vi "LogToFile.vi"(0 "EventData in":T1, 11 "Error In":errorcluster) -> (4 "EventData out":T1, 15 "Error Out":errorcluster)   [LabVIEW 2021, in "Event Logger.lvlib"]
uses:
  Event Logger.lvlib
  TypeDef/EventDataCluster.ctl
  TypeDef/EventValues.ctl
  Migrator/Migrator Reusables/Migrator Reusables.lvlib
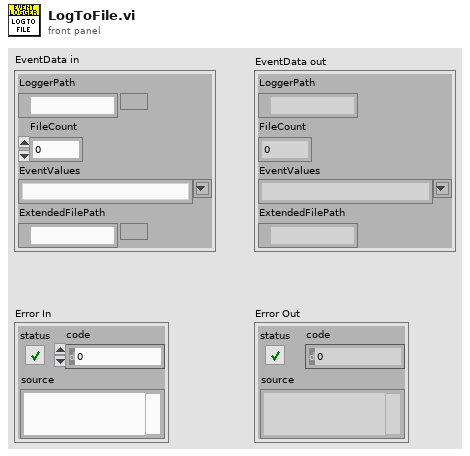
[diagram p1: front panel]
types:
  T1 = typedef "Event Logger.lvlib/EventDataCluster.ctl" = cluster{"LoggerPath":path, "FileCount":i32, "EventValues":T2, "ExtendedFilePath":path}
  T2 = typedef "Event Logger.lvlib/EventValues.ctl" = string
  T3 = typedef "Migrator Reusables.lvlib/ErrorInformation.ctl" = cluster{"Subroutine":string, "ErrorData":errorcluster}
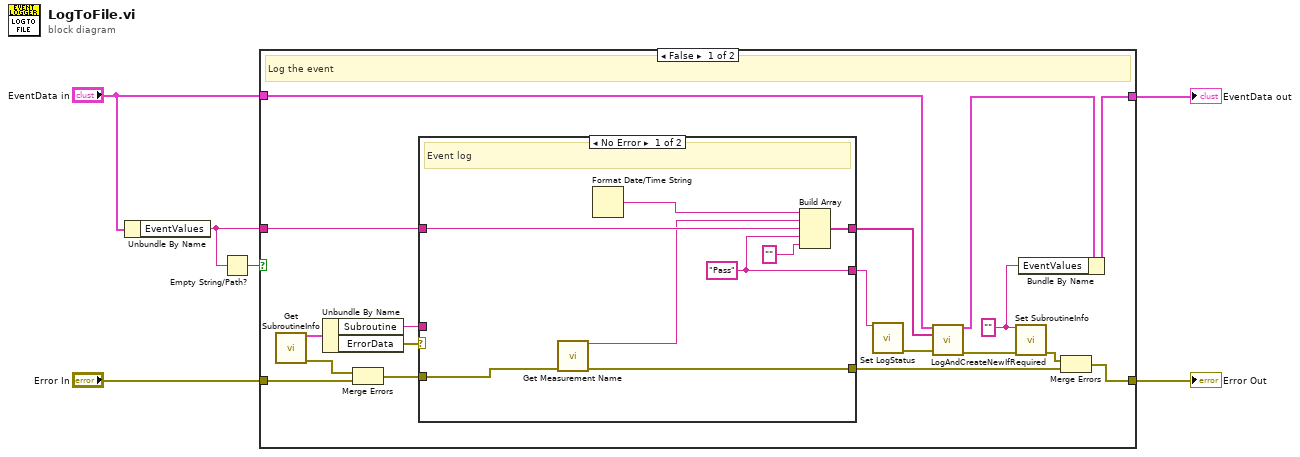
[diagram p0: block diagram]
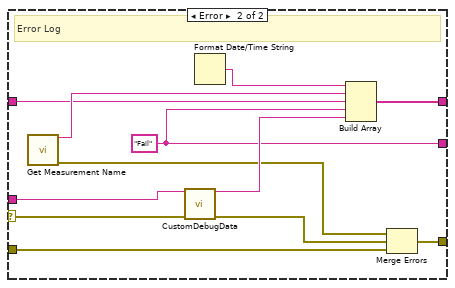
[diagram p2: hidden frame]
diagram:
  n1 = Unbundle By Name("EventData in") -> ("EventValues"=w2:T2)
  n2 = Empty String/Path?(string/path=w2) -> (empty?=w1:bool)
  n3 = case shown="False" w1 {
    tunnel: "Error In" -> [w24 w45]
    tunnel: [w23 w45] -> w5
    tunnel: "EventData in" -> [w10 w46]
    tunnel: w2 -> [w9 _]
    tunnel: [w8 w46] -> w3
    frame False {
      w7 = "" ("Subroutine In")
      # "Log the event"
      n4 = call "Get SubroutineInfo.vi"() -> ("data"=w22:T3, "error out"=w20:errorcluster)  [unwired: 14 in]
      n5 = Unbundle By Name(w22) -> ("Subroutine"=w17:string, "ErrorData"=w19:errorcluster)
      n6 = Merge Errors(w20, w24) -> (w21:errorcluster)
      n7 = case shown="No Error" w19 {
        selector: w19 -> [_ w39]
        tunnel: w9 -> [w32 w42]
        tunnel: w21 -> [w31 w38]
        tunnel: [w28 w40] -> w14
        tunnel: [w30 w41] -> w18
        tunnel: w17 -> [_ w36]
        tunnel: [w27 w35] -> w12
        frame No Error {
          w27 = "Pass" ("StatusIn")
          # "Event log"
          n8 = call "Get Measurement Name.vi"("error in (no error)"=w31) -> ("Name Out"=w29:string, "error out"=w28:errorcluster)  [unwired: 13 in]
          n9 = Format Date/Time String() -> (date/time string=w25:string)  [unwired: 3 in]
          n10 = Build Array(w25, w29, w32, w27, "") -> (w30:T2[])
        }
        frame Error {
          w35 = "Fail" ("StatusIn")
          # "Error Log"
          n11 = call "Get Measurement Name.vi"() -> ("Name Out"=w44:string, "error out"=w34:errorcluster)  [unwired: 14 in]
          n12 = call "CustomDebugData.vi"("Subroutine"=w36, "error in (no error)"=w39) -> ("DebugInfo"=w43:string, "error out"=w37:errorcluster)  [unwired: 12 in]
          n13 = Format Date/Time String() -> (date/time string=w33:string)  [unwired: 3 in]
          n14 = Build Array(w33, w44, w42, w35, w43) -> (w41:T2[])
          n15 = Merge Errors(w34, w37, w38) -> (w40:errorcluster)
        }
      }
      n16 = call "Set LogStatus.vi"("StatusIn"=w12) -> ("error out"=w13:errorcluster)  [unwired: 14 in]
      n17 = call "LogAndCreateNewIfRequired.vi"("EventData in"=w10, "LogDataIn"=w18, "error in (no error)"=w13) -> ("EventData out"=w11:T1, "error out"=w16:errorcluster)  [unwired: 11 in]
      n18 = call "Set SubroutineInfo.vi"("Subroutine In"=w7, "error in (no error)"=w16) -> ("error out"=w15:errorcluster)  [unwired: 13 in]
      n19 = Bundle By Name(cluster=w11, "EventValues"=w7) -> (w8:T1)
      n20 = Merge Errors(w15, w14) -> (w23:errorcluster)
    }
    frame True {
      # "Skip logging activity if the event value is empty"
    }
  }
  "Error Out" <- w5
  "EventData out" <- w3
